vi "Prober_ProbeTouchdown.vi"(8 "error in (no error)":errorcluster, 11 "ProbeStationControl in":refnum<class "ProbeStationControl.lvclass">) -> (0 "error out":errorcluster, 1 "previous Z [µm]":i32, 2 "Z [µm]":i32, 3 "ProbeStationControl out":refnum<class "ProbeStationControl.lvclass">)   [LabVIEW 2013, in "ProbeStationControl.lvclass"]
uses:
  ProbeStationControl.lvclass
  ProbeStationControl.lvclass/ProbeStationControl.ctl
  InstrumentSetup.vi
  <vilib>/Utility/error.llb/Error Cluster From Error Code.vi
  <vilib>/ErrorRing/Error Ring.xnode
  ArduinoControl/ArduinoControl.lvclass
  InstrControl.lvclass
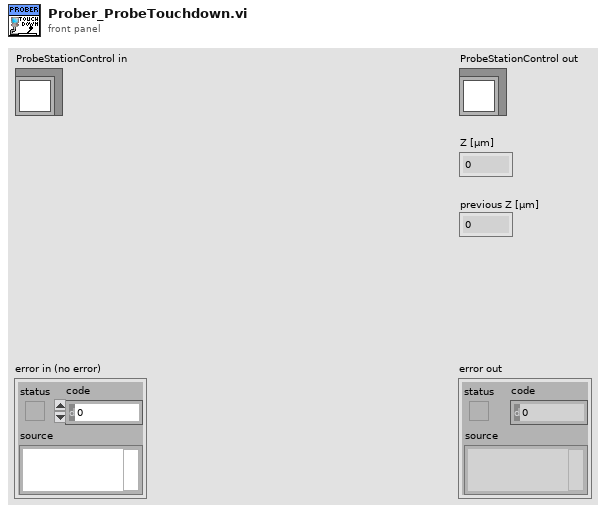
[diagram p1: front panel]
types:
  T1 = cluster{"touchdown height [µm]":i32, "search band [µm]":u32, "speed [µm/step]":u32, "overdrive [µm]":u32}
  T2 = cluster{"VISA address":refnum<visa-resource-name>, "T sensor":enum16{"SHT", "DS"}, "Arduino":refnum<class "ArduinoControl.lvclass">}
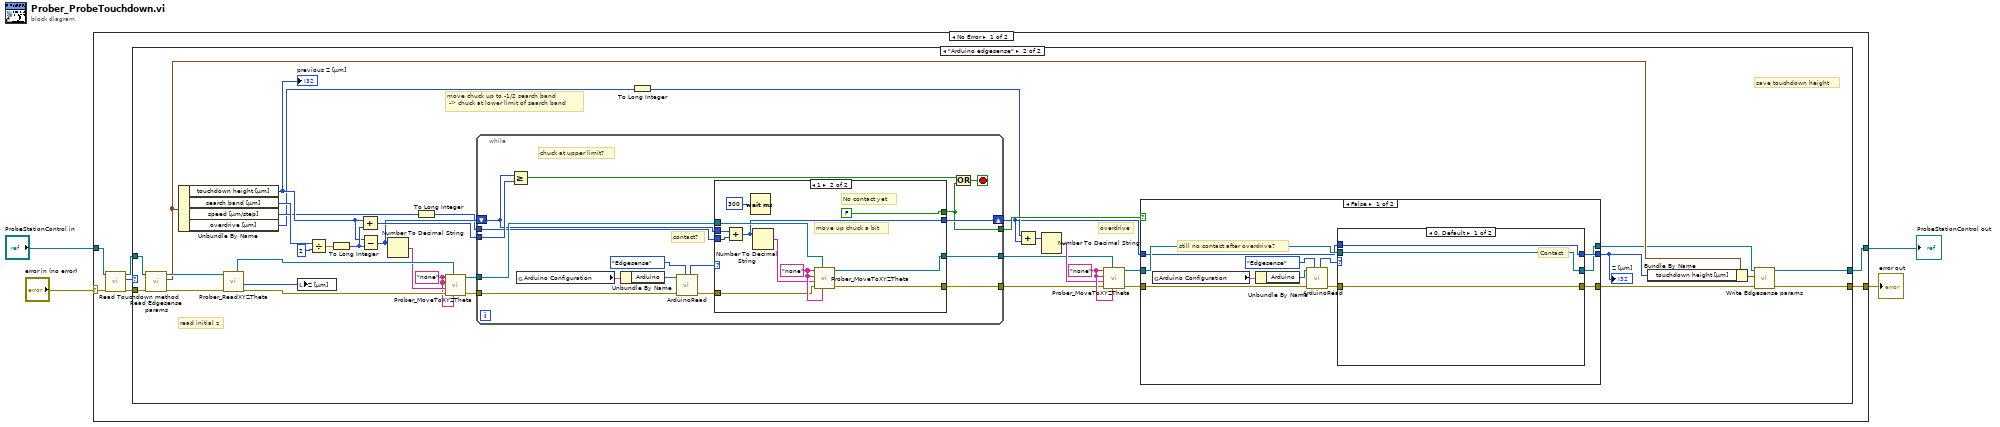
[diagram p0: block diagram]
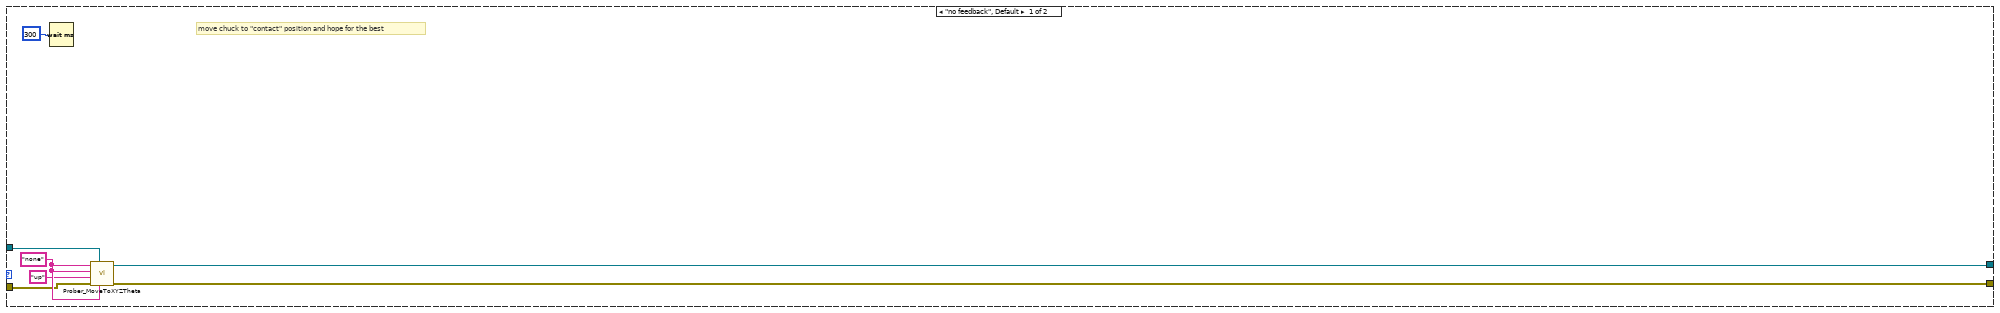
[diagram p2: hidden frame]
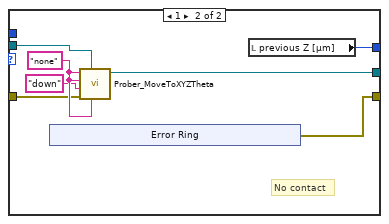
[diagram p3: hidden frame]
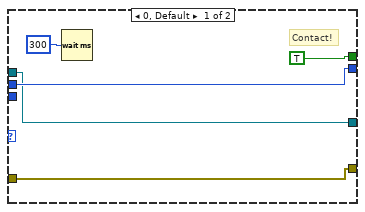
[diagram p5: hidden frame]
diagram:
  n1 = case shown="No Error" "error in (no error)" {
    selector: "error in (no error)" -> [w9 w119]
    tunnel: [w11 w119] -> w3
    tunnel: [w10 w118] -> w1
    tunnel: "ProbeStationControl in" -> [w7 w118]
    frame No Error {
      n2 = call "Read Touchdown method.vi"("error in (no error)"=w9, "ProbeStationControl in"=w7) -> ("error out"=w8:errorcluster, "Touchdown method"=w5:enum16{"no feedback", "Arduino edgesense"}, "ProbeStationControl out"=w6:refnum<class "ProbeStationControl.lvclass">)  [unwired: 7 in]
      n3 = case shown="\"Arduino edgesense\"" w5 {
        tunnel: w6 -> [w15 w56]
        tunnel: w8 -> [w14 w55]
        tunnel: [w12 w20] -> w11
        tunnel: [w13 w19] -> w10
        frame "no feedback", Default {
          w17 = "none"
          # "move chuck to \"contact\" position and hope for the best"
          n4 = Wait (ms)(milliseconds to wait=300) -> ()  [unwired: 1 out]
          n5 = call "Prober_MoveToXYZTheta.vi"("Theta location [mdeg]"=w17, "ProbeStationControl in"=w15, "error in (no error)"=w14, "Z location [µm]"="up", "Y location [µm]"=w17, "X location [µm]"=w17) -> ("error out"=w12:errorcluster, "ProbeStationControl out"=w13:refnum<class "ProbeStationControl.lvclass">)  [unwired: 3 in, 1 out]
        }
        frame "Arduino edgesense" {
          w35 = "none" ("Z location")
          w41 = "none" ("Z location")
          # "save touchdown height"
          # "overdrive"
          # "move chuck up to -1/2 search band\n -> chuck at lower limit of search band"
          # "read initial z"
          n6 = call "Read Edgesense params.vi"("error in (no error)"=w55, "ProbeStationControl in"=w56) -> ("error out"=w43:errorcluster, "Edgesense params"=w23:T1, "ProbeStationControl out"=w54:refnum<class "ProbeStationControl.lvclass">)  [unwired: 7 in]
          n7 = Unbundle By Name(w23) -> ("touchdown height [µm]"=w45:i32, "search band [µm]"=w48:u32, "speed [µm/step]"=w38:u32, "overdrive [µm]"=w28:u32)
          "previous Z [µm]" <- w45
          n8 = call "Prober_ReadXYZTheta.vi"("error in (no error)"=w43, "ProbeStationControl in"=w54) -> ("error out"=w52:errorcluster, "Z location [µm]"=w50:i32, "ProbeStationControl out"=w51:refnum<class "ProbeStationControl.lvclass">)  [unwired: 4 in, 3 out]
          n9 = local write "Z [µm]"(w50) -> ()
          n10 = Divide(x=w48, y=u32 2) -> (x/y=w47:dbl)
          n11 = To Long Integer(number=w47) -> (32bit integer=w46:i32)
          n12 = Add(x=w45, y=w46) -> (x+y=w44:i32)
          n13 = Subtract(x=w45, y=w46) -> (x-y=w39:i32)
          n14 = Number To Decimal String(number=w39) -> (decimal integer string=w49:string)  [unwired: 1 in]
          n15 = To Long Integer(number=w38) -> (32bit integer=w37:i32)
          n16 = call "Prober_MoveToXYZTheta.vi"("Theta location [mdeg]"=w41, "ProbeStationControl in"=w51, "error in (no error)"=w52, "Z location [µm]"=w49, "Y location [µm]"=w41, "X location [µm]"=w41) -> ("error out"=w42:errorcluster, "ProbeStationControl out"=w40:refnum<class "ProbeStationControl.lvclass">)  [unwired: 3 in, 1 out]
          n17 = while {
            tunnel: w44 -> [w101]
            shift-right: [w88] -> w25
            shift-left: w39 -> [w89]
            tunnel: w42 -> [w99]
            tunnel: w37 -> [w87]
            tunnel: w40 -> [w92]
            tunnel: [w91] -> w31
            tunnel: [w90] -> w32
            tunnel: [w86] -> w36
            stop <- w95 stop-if-true
            # "contact?"
            # "chuck at upper limit?"
            n18 = Greater Or Equal?(x=w89, y=w101) -> (x >= y?=w94:bool)
            n19 = global read "InstrumentSetup.vi" "Arduino Configuration"() -> (w98:T2)
            n20 = Unbundle By Name(w98) -> ("Arduino"=w97:refnum<class "ArduinoControl.lvclass">)
            n21 = call "ArduinoRead.vi"("Arduino function"=enum16{"T/RH", "Interlock", "Edgesense"}."Edgesense", "error in (no error)"=w99, "ArduinoControl in"=w97) -> ("error out"=w93:errorcluster, "Edgesense Status"=w96:u16)  [unwired: 3 in, 4 out]
            n22 = case shown="1" w96 {
              tunnel: w87 -> [_ w117]
              tunnel: w89 -> [w103 w108]
              tunnel: [w103 w107] -> w88
              tunnel: [TRUE FALSE] -> w86
              tunnel: w93 -> [w105 w113]
              tunnel: [w105 w112] -> w90
              tunnel: w92 -> [w102 w110]
              tunnel: [w102 w109] -> w91
              frame 0, Default {
                # "Contact!"
                n23 = Wait (ms)(milliseconds to wait=300) -> ()  [unwired: 1 out]
              }
              frame 1 {
                w115 = "none" ("Z location")
                # "move up chuck a bit"
                # "No contact yet"
                n24 = Add(x=w108, y=w117) -> (x+y=w107:i32)
                n25 = Wait (ms)(milliseconds to wait=300) -> ()  [unwired: 1 out]
                n26 = Number To Decimal String(number=w107) -> (decimal integer string=w114:string)  [unwired: 1 in]
                n27 = call "Prober_MoveToXYZTheta.vi"("Theta location [mdeg]"=w115, "ProbeStationControl in"=w110, "error in (no error)"=w113, "Z location [µm]"=w114, "Y location [µm]"=w115, "X location [µm]"=w115) -> ("error out"=w112:errorcluster, "ProbeStationControl out"=w109:refnum<class "ProbeStationControl.lvclass">)  [unwired: 3 in, 1 out]
              }
            }
            n28 = Or(x=w94, y=w86) -> (x .or. y?=w95:bool)
          }
          n29 = To Long Integer(number=w28) -> (32bit integer=w27:i32)
          n30 = Add(x=w27, y=w25) -> (x+y=w34:i32)
          n31 = Number To Decimal String(number=w34) -> (decimal integer string=w33:string)  [unwired: 1 in]
          n32 = call "Prober_MoveToXYZTheta.vi"("Theta location [mdeg]"=w35, "ProbeStationControl in"=w31, "error in (no error)"=w32, "Z location [µm]"=w33, "Y location [µm]"=w35, "X location [µm]"=w35) -> ("error out"=w30:errorcluster, "ProbeStationControl out"=w29:refnum<class "ProbeStationControl.lvclass">)  [unwired: 3 in, 1 out]
          n33 = case shown="False" w36 {
            tunnel: w30 -> [w64 w83]
            tunnel: w29 -> [w62 w84]
            tunnel: w25 -> [w60 w85]
            tunnel: [w59 w85] -> w24
            tunnel: [w58 w84] -> w22
            tunnel: [w57 w83] -> w21
            frame False {
              # "still no contact after overdrive?"
              n34 = global read "InstrumentSetup.vi" "Arduino Configuration"() -> (w66:T2)
              n35 = Unbundle By Name(w66) -> ("Arduino"=w67:refnum<class "ArduinoControl.lvclass">)
              n36 = call "ArduinoRead.vi"("Arduino function"=enum16{"T/RH", "Interlock", "Edgesense"}."Edgesense", "error in (no error)"=w64, "ArduinoControl in"=w67) -> ("error out"=w61:errorcluster, "Edgesense Status"=w63:u16)  [unwired: 3 in, 4 out]
              n37 = case shown="0, Default" w63 {
                tunnel: w62 -> [w69 w74]
                tunnel: w61 -> [w68 w73]
                tunnel: w60 -> [w70 _]
                tunnel: [w70 w77] -> w59
                tunnel: [w69 w72] -> w58
                tunnel: [w68 w71] -> w57
                frame 0, Default {
                  # "Contact"
                }
                frame 1 {
                  w76 = "none" ("Z location")
                  # "No contact"
                  n38 = xnode "Error Ring"() -> ("error out"=w71:errorcluster)
                  n39 = call "Prober_MoveToXYZTheta.vi"("Theta location [mdeg]"=w76, "ProbeStationControl in"=w74, "error in (no error)"=w73, "Z location [µm]"="down", "Y location [µm]"=w76, "X location [µm]"=w76) -> ("ProbeStationControl out"=w72:refnum<class "ProbeStationControl.lvclass">)  [unwired: 3 in, 2 out]
                  n40 = local read "previous Z [µm]"() -> (w77:i32)
                }
              }
            }
            frame True {
            }
          }
          "Z [µm]" <- w24
          n41 = Bundle By Name(cluster=w23, "touchdown height [µm]"=w24) -> (w26:T1)
          n42 = call "Write Edgesense params.vi"("error in (no error)"=w21, "Edgesense params"=w26, "ProbeStationControl in"=w22) -> ("error out"=w20:errorcluster, "ProbeStationControl out"=w19:refnum<class "ProbeStationControl.lvclass">)  [unwired: 7 in]
        }
      }
    }
    frame Error {
    }
  }
  "error out" <- w3
  "ProbeStationControl out" <- w1
